vi "Insert Element at End.vi"(8 "error in (no error)":errorcluster, 9 "element":variant, 10 "Name":string, 11 "Variant in":variant) -> (0 "error out":errorcluster, 3 "Variant out":variant)   [LabVIEW 2017, in "Advanced Variant Tools.lvlib" / "Data Manipulation.lvlib"]
uses:
  Data Manipulation.lvlib
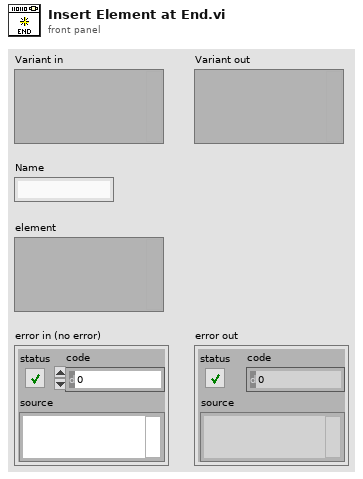
[diagram p1: front panel]
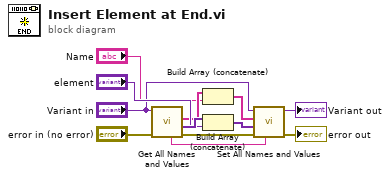
[diagram p0: block diagram]
diagram:
  n1 = call "Get All Names and Values.vi"("error in"="error in (no error)", "Cluster In"="Variant in") -> ("error out"=w10:errorcluster, "Values"=w11:variant[], "Item Names"=w4:string[], "Name"=w1:string)  [unwired: 5 in, 1 out]
  n2 = Build Array (concatenate)(w4, "Name") -> (w2:string[])
  n3 = Build Array (concatenate)(w11, "element") -> (w7:variant[])
  n4 = call "Set All Names and Values.vi"("Name"=w1, "error in"=w10, "values"=w7, "Item Names"=w2, "Cluster In"="Variant in") -> ("error out"=→"error out":errorcluster, "Cluster Out"=→"Variant out":variant)  [unwired: 5 in]
